vi "testProcessCmd.vi"(8 "error in (no error)":errorcluster) -> (0 "error out":errorcluster)   [LabVIEW 2018]
doc: "Test the processCmd.vi."
uses:
  src/TcpServer/TcpServer.lvclass
  src/TcpServer/TcpServer.lvclass/TcpServer.ctl
  src/TcpServer/typedef/tcpPacketTypeDef.ctl
  <vilib>/addons/_JKI Toolkits/Caraya/classes/Assert/Assert Equal Value_Variant.vi
  <vilib>/addons/_JKI Toolkits/Caraya/classes/Test/Test.lvclass
  <vilib>/addons/_JKI Toolkits/Caraya/classes/Assert/Assert.lvclass
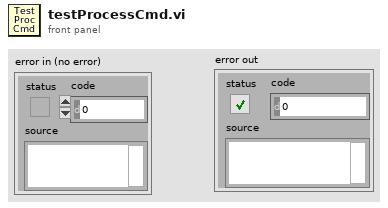
[diagram p1: front panel]
types:
  T1 = typedef "TcpServer.lvclass/tcpPacketTypeDef.ctl" = cluster{"packet":string, "firstPacket":bool, "firstConnection":bool}
  T2 = typedef "TcpServer.lvclass/packetConnIDTypeDef.ctl" = cluster{"packet":string, "firstPacket":bool, "firstConnection":bool}
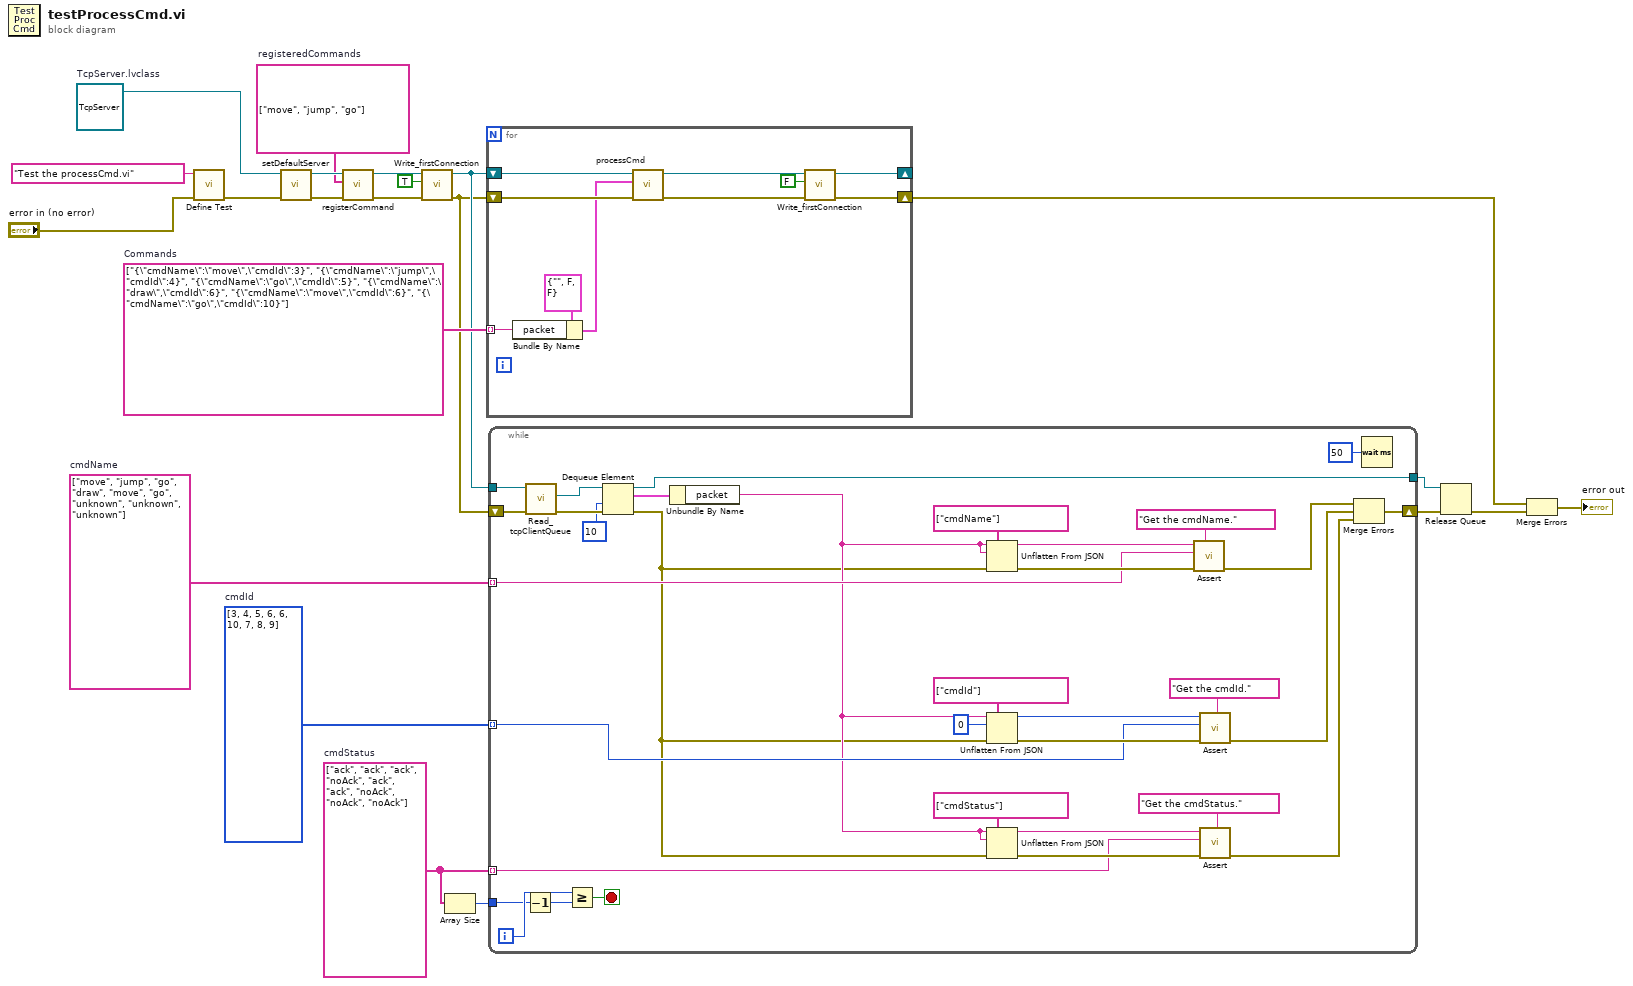
[diagram p0: block diagram]
diagram:
  w6 = string[] ["ack", "ack", "ack", "noAck", "ack", "ack", "noAck", "noAck", "noAck"]  # cmdStatus
  w7 = i32[] [3, 4, 5, 6, 6, 10, 7, 8, 9]  # cmdId
  w8 = string[] ["move", "jump", "go", "draw", "move", "go", "unknown", "unknown", "unknown"]  # cmdName
  w14 = string[] ["{\"cmdName\":\"move\",\"cmdId\":3}", "{\"cmdName\":\"jump\",\"cmdId\":4}", "{\"cmdName\":\"go\",\"cmdId\":5}", "{\"cmdName\":\"draw\",\"cmdId\":6}", "{\"cmdName\":\"move\",\"cmdId\":6}", "{\"cmdName\":\"go\",\"cmdId\":10}"]  # Commands
  w15 = string[] ["move", "jump", "go"]  # registeredCommands
  w19 = refnum<class "TcpServer.lvclass"> refnum  # TcpServer.lvclass
  n1 = call <vilib>:"Define Test.vi"("error in (no error)"="error in (no error)", "Label (VI Title)"="Test the processCmd.vi") -> ("error out"=w21:errorcluster)  [unwired: 9 in]
  n2 = call "setDefaultServer.vi"("error in (no error)"=w21, "TcpServer.lvclass"=w19) -> ("error out"=w17:errorcluster, "tcpServer out"=w16:refnum<class "TcpServer.lvclass">)  [unwired: 8 in]
  n3 = call "registerCommand.vi"("error in (no error)"=w17, "registeredCommands"=w15, "tcpServer in"=w16) -> ("error out"=w18:errorcluster, "tcpServer out"=w13:refnum<class "TcpServer.lvclass">)  [unwired: 7 in]
  n4 = call "Write_firstConnection.vi"("error in (no error)"=w18, "firstConnection"=TRUE, "TcpServer in"=w13) -> ("error out"=w9:errorcluster, "TcpServer out"=w10:refnum<class "TcpServer.lvclass">)  [unwired: 7 in]
  n5 = Array Size(array=w6) -> (size(s)=w5:i32)
  n6 = for {
    tunnel: w14 -> [w28] mode=indexing
    shift-right: [w24] -> _
    shift-left: w10 -> [w30]
    shift-right: [w26] -> w4
    shift-left: w9 -> [w32]
    n7 = Bundle By Name(cluster=T1 {"packet"="", "firstPacket"=FALSE, "firstConnection"=FALSE} ("packetConnID"), "packet"=w28) -> (w29:T1)
    n8 = call "processCmd.vi"("error in (no error)"=w32, "tcpPacket"=w29, "tcpServer in"=w30) -> ("error out"=w27:errorcluster, "tcpServer out"=w25:refnum<class "TcpServer.lvclass">)  [unwired: 7 in]
    n9 = call "Write_firstConnection.vi"("error in (no error)"=w27, "firstConnection"=FALSE, "TcpServer in"=w25) -> ("error out"=w26:errorcluster, "TcpServer out"=w24:refnum<class "TcpServer.lvclass">)  [unwired: 7 in]
  }
  n10 = while {
    tunnel: w10 -> [w63]
    tunnel: w8 -> [w52] mode=indexing
    tunnel: w7 -> [w46] mode=indexing
    tunnel: w6 -> [w45] mode=indexing
    tunnel: w5 -> [w40]
    shift-right: [w34] -> w3
    shift-left: w9 -> [w62]
    tunnel: [w33] -> w1
    i -> [w41]
    stop <- w42 stop-if-true
    n11 = Decrement(x=w40) -> (x-1=w39:i32)
    n12 = call "Read_tcpClientQueue.vi"("error in (no error)"=w62, "tcpServer in"=w63) -> ("error out"=w65:errorcluster, "tcpClientQueue"=w64:refnum<queue>)  [unwired: 7 in, 1 out]
    n13 = Greater Or Equal?(x=w41, y=w39) -> (x >= y?=w42:bool)
    n14 = Dequeue Element(queue=w64, timeout in ms (-1)=10, error in (no error)=w65) -> (queue out=w33:refnum<queue>, element=w66:T2, error out=w38:errorcluster)  [unwired: 1 out]
    n15 = Unbundle By Name(w66) -> ("packet"=w44:string)
    n16 = Unflatten From JSON(path=string[] ["cmdName"], JSON string=w44, type and defaults=w44, error in (no error)=w38) -> (value=w59:string, error out=w56:errorcluster)  [unwired: 3 in]
    n17 = Unflatten From JSON(path=string[] ["cmdId"], JSON string=w44, type and defaults=0, error in (no error)=w38) -> (value=w60:i32, error out=w55:errorcluster)  [unwired: 3 in]
    n18 = Unflatten From JSON(path=string[] ["cmdStatus"], JSON string=w44, type and defaults=w44, error in (no error)=w38) -> (value=w48:string, error out=w50:errorcluster)  [unwired: 3 in]
    n19 = call-poly <vilib>:"Assert.vi"("Label"="Get the cmdName.", "error in (no error)"=w56, "Y"=w52, "X"=w59) -> ("error out"=w37:errorcluster)  [unwired: 7 in]
    n20 = call-poly <vilib>:"Assert.vi"("Label"="Get the cmdId.", "error in (no error)"=w55, "Y"=w46, "X"=w60) -> ("error out"=w36:errorcluster)  [unwired: 7 in]
    n21 = call-poly <vilib>:"Assert.vi"("Label"="Get the cmdStatus.", "error in (no error)"=w50, "Y"=w45, "X"=w48) -> ("error out"=w35:errorcluster)  [unwired: 7 in]
    n22 = Merge Errors(w37, w36, w35) -> (w34:errorcluster)
    n23 = Wait (ms)(milliseconds to wait=u32 50) -> ()  [unwired: 1 out]
  }
  n24 = Release Queue(queue=w1, error in (no error)=w3) -> (error out=w2:errorcluster)  [unwired: 1 in, 2 out]
  n25 = Merge Errors(w4, w2) -> (→"error out":errorcluster)
